vi "Get Public Registry Events.vi"(8 "error in (no error)":errorcluster) -> (0 "error out":errorcluster, 3 "Public Registry Events":T1)   [LabVIEW 2019, in "Registry-SMO.lvclass"]
doc: "JKI State Machine Objects (SMO) 1.3.0.56\nJKI - JKI\nCopyright (c) 2017, JKI"
uses:
  Registry-SMO.lvclass
  PublicRegistryEvents--Cluster.ctl
  SMO_Info--Cluster.ctl
  Registry-SMO.lvclass/Registry-SMO.ctl
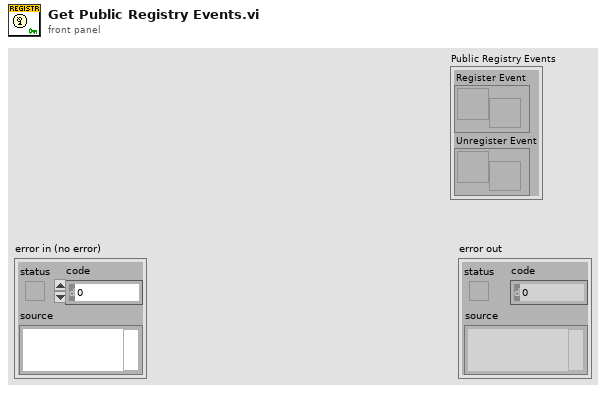
[diagram p1: front panel]
types:
  T1 = typedef "Registry-SMO.lvclass/PublicRegistryEvents--Cluster.ctl" = cluster{"Register Event":refnum<user-event>, "Unregister Event":refnum<user-event>}
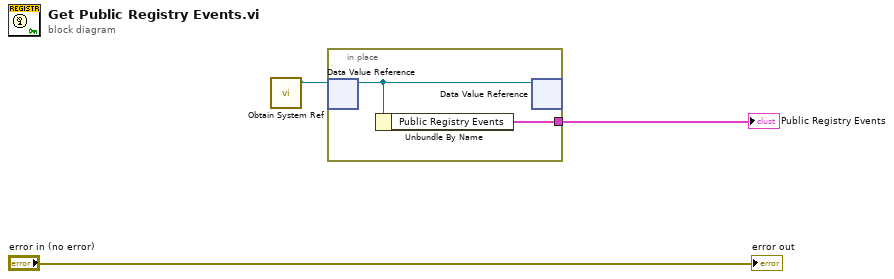
[diagram p0: block diagram]
diagram:
  n1 = call "Obtain System Ref.vi"() -> ("JKI SMO System"=w2:refnum<data-value>)  [unwired: 10 in, 1 out]
  n2 = in-place {
    in-place-border: [w4] -> w1
    n3 = in-place-dvr #1(w2) -> (w5:refnum<class "Registry-SMO.lvclass">)  [unwired: 1 out]
    n4 = Unbundle By Name(w5) -> ("Public Registry Events"=w4:T1)
    n5 = in-place-dvr #1(w5) -> ()  [unwired: 2 out]
  }
  "Public Registry Events" <- w1
  "error out" <- "error in (no error)"
